vi "Fetch Logged Data.vi"(8 "error in (no error)":errorcluster, 9 "Reading Count (0)":i32, 10 "Channel (1)":string="1", 11 "VISA resource name":refnum<visa-resource-name>) -> (0 "error out":errorcluster, 2 "Logged Data":dbl[](array[numeric]), 3 "VISA resource name out":refnum<visa-resource-name>)   [LabVIEW 2020, in "Keysight E36300 Series.lvlib"]
doc: "Fetches numbers of logged data from the channels.\n\n<b>Note: </b>\n(1)This VI is only applicable for E36312A and E36313A models.\n(2)Must start the data logger by <b>Start Data Logger</b> VI before fetch logger data.\n(3)Uses <b>Stop Data Logger</b> VI to stop data logger after fetch logger data."
uses:
  Keysight E36300 Series.lvlib
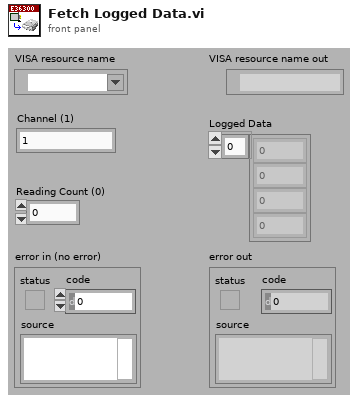
[diagram p1: front panel]
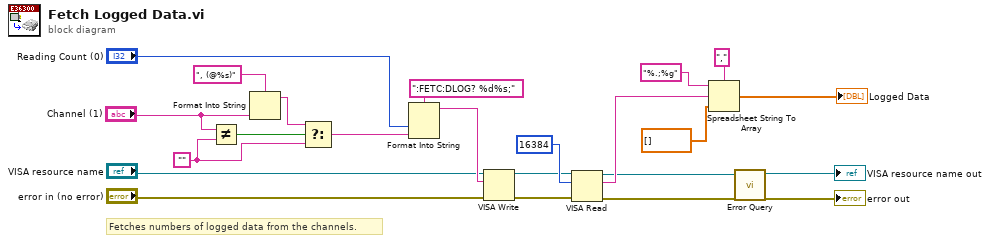
[diagram p0: block diagram]
diagram:
  w3 = ""
  # "Fetches numbers of logged data from the channels."
  n1 = Not Equal?(x="Channel (1)", y=w3) -> (x != y?=w4:bool)
  n2 = Format Into String(format string=", (@%s)", "Channel (1)") -> (resulting string=w5:string)  [unwired: 2 in, 1 out]
  n3 = Select(t=w5, s=w4, f=w3) -> (s? t:f=w1:string)
  n4 = Format Into String(format string=":FETC:DLOG? %d%s;", "Reading Count (0)", w1) -> (resulting string=w21:string)  [unwired: 2 in, 1 out]
  n5 = VISA Write(VISA resource name="VISA resource name", write buffer=w21, error in (no error)="error in (no error)") -> (VISA resource name out=w11:refnum<visa-resource-name>, error out=w10:errorcluster)  [unwired: 1 out]
  n6 = VISA Read(VISA resource name=w11, byte count=u32 16384, error in (no error)=w10) -> (VISA resource name out=w9:refnum<visa-resource-name>, read buffer=w15:string, error out=w8:errorcluster)  [unwired: 1 out]
  n7 = Spreadsheet String To Array(delimiter (Tab)=",", format string="%.;%g", spreadsheet string=w15, array type (2D Dbl)=dbl[] []) -> (array=→"Logged Data":dbl[])
  n8 = call "Error Query.vi"("error in (no error)"=w8, "VISA resource name"=w9) -> ("error out"=→"error out":errorcluster, "VISA resource name out"=→"VISA resource name out":refnum<visa-resource-name>)  [unwired: 6 in, 2 out]
